vi "Dashboard Application.vi"   [LabVIEW 2019]
uses:
  Dashboard/Dashboard.lvclass
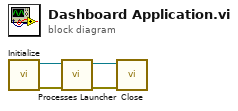
[diagram p0: block diagram]
diagram:
  n1 = call "Initialize.vi"() -> ("Error Out"=w3:errorcluster, "Dashboard"=w4:refnum<class "Dashboard.lvclass">)  [unwired: 10 in]
  n2 = call "Processes Launcher.vi"("Error In"=w3, "Dashboard In"=w4) -> ("Error Out"=w1:errorcluster, "Dashboard Out"=w2:refnum<class "Dashboard.lvclass">)  [unwired: 8 in]
  n3 = call "Close.vi"("Error In"=w1, "Dashboard"=w2) -> ()  [unwired: 9 in, 1 out]
